vi "IniConfigData.vi"(11 "Enum":T1=enum."Read Key") -> ()   [LabVIEW 2014]
uses:
  ReadWriteIniKey.ctl
  Robot Global Data.vi
  <vilib>/Utility/config.llb/NI_LVConfig.lvlib
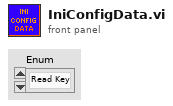
[diagram p1: front panel]
types:
  T1 = typedef "ReadWriteIniKey.ctl" = enum16{"Write Key", "Read Key"}
  T2 = typedef "NI_LVConfig.lvlib/Config Data RefNum.ctl" = refnum<k1>
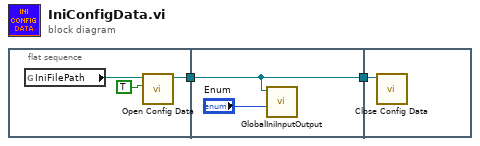
[diagram p0: block diagram]
diagram:
  n1 = flat-sequence {
    tunnel: [w3] -> w1
    tunnel: [w7] -> w2
    tunnel: w1 -> [w7]
    tunnel: w2 -> [w8]
    frame #0 {
      n2 = global read "Robot Global Data.vi" "IniFilePath"() -> (w5:path)
      n3 = call <vilib>:"Open Config Data.vi"("create file if necessary (T)"=TRUE, "configuration file path"=w5) -> ("refnum"=w3:T2)  [unwired: 7 in, 2 out]
    }
    frame #1 {
      n4 = call "GlobalIniInputOutput.vi"("Read or Write"="Enum", "Ini File Refnum"=w7) -> ()  [unwired: 10 in]
    }
    frame #2 {
      n5 = call <vilib>:"Close Config Data.vi"("refnum"=w8) -> ()  [unwired: 9 in, 2 out]
    }
  }
